vi "WinHostToFlexRIO.vi"() -> ()   [LabVIEW 2013]
doc: "This is the host VI for the 10-Tap 8-Bit Camera with DRAM example. This example demonstrates how to acquire images from a 10-tap, 8-bit, extended configuration, Camera Link camera and display the images on the host. This example supports area scan and line scan cameras for both continuous and finite acquisitions.\n\nThis example also demonstrates the use of DRAM as a frame buffer for very high speed acquisitions. Data packing and flow-control are also employed to maximize use of the available DRAM and FIFOs in terms of both memory space and performance.\n\nAdditionally, the example demonstrates the serial server, which allows third-party camera configuration utilities to communicate with the camera using the Camera Link serial interface while this VI is running."
uses:
  <vilib>/userdefined/High Color/nirio_resource_hc.ctl
  <vilib>/FPGAPlugInAG/PXIe-7966R/niLvFpga_Open_PXIe-7966R.vi
  <vilib>/rvi/interface/common/dynamic/niFpgaDynamicAddResources.vi
  <vilib>/FPGAPlugInAG/Dynamic/niLvFpga_Reset_Dynamic.vi
  <vilib>/rvi/interface/common/niFpgaWaitOnOcc.vi
  <vilib>/Utility/error.llb/Error Cluster From Error Code.vi
  <vilib>/rvi/errors/niLvFpgaAdjustHostInterfaceError.vi
  <vilib>/FPGAPlugInAG/Dynamic/niLvFpga_Run_Dynamic.vi
  <vilib>/LabVIEW Targets/FPGA/FlexRIO/CustomFPGAMethods/79XXR_Method_IOModuleStatusImpl.vi
  <vilib>/FPGAPlugInAG/Dynamic/niLvFpga_Close_Dynamic.vi
  <vilib>/rvi/interface/nirviOpenFPGA/nirviOpenFPGA.xnode
  FPGA Bitfiles/PXIe-7966R_FlexRIOMod1483_8T8_v1_0.lvbitx
  FlexRIO1483_8T8.vi
  <vilib>/rvi/interface/nirviMethod/nirviMethod.xnode
  <vilib>/rvi/interface/nirviReadWriteControl/nirviReadWriteControl.xnode
  <vilib>/rvi/interface/nirviCloseFPGA/nirviCloseFPGA.xnode
  <vilib>/rvi/interface/Simulation/niFpgaSimulationCallBeginRW.vi
  <vilib>/rvi/errors/niLvFpgaMergeErrorWithErrorCode.vi
  <vilib>/FPGAPlugInAG/Dynamic/niLvFpga_ReadFifo_Dynamic.vi
  NiFpgaLv.dll
  <vilib>/FPGAPlugInAG/Dynamic/niLvFpga_ConfigureFifo_Dynamic.vi
  <vilib>/FPGAPlugInAG/Dynamic/niLvFpga_StartFifo_Dynamic.vi
panel:
  out "Frames Received":u32
  out "Error out":errorcluster
  out "Received":bool
  out "Sent":bool
  out "Acquire 3":bool
  out "UART  Received Message":string
  in  "Acquire 2":bool
  in  "UART  Send Message":string
  out "Frame Counter Check":bool
  in  "RIO Device":T1="RIO0"
  out "Ready":bool
  out "Image":T2(plugin-control)
  in  "DAQStartStop":bool
  in  "Stop":bool
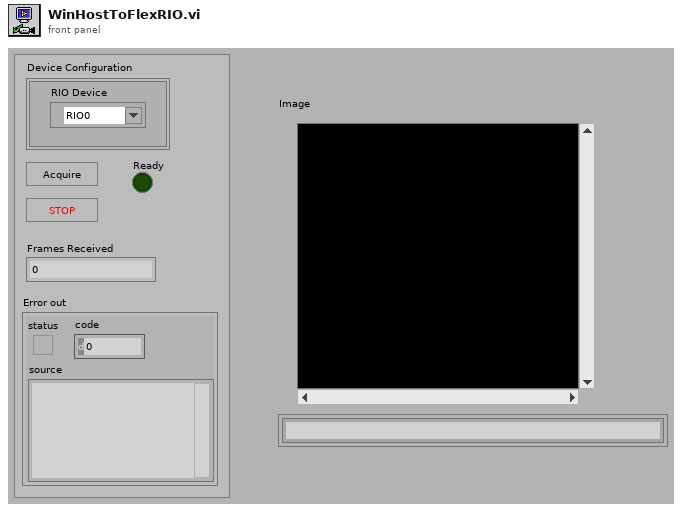
[diagram p1: front panel]
types:
  T1 = typedef "nirio_resource_hc.ctl" = tag
  T2 = typedef "IMAQ Image.ctl" = refnum<image>
  T3 = enum8{"Standard", "Basler 10-tap", "Vosskühler 10-tap"}
  T4 = typedef "Image Type" = u32
  T5 = enum16{"big-endian, network order", "native, host order", "little-endian"}
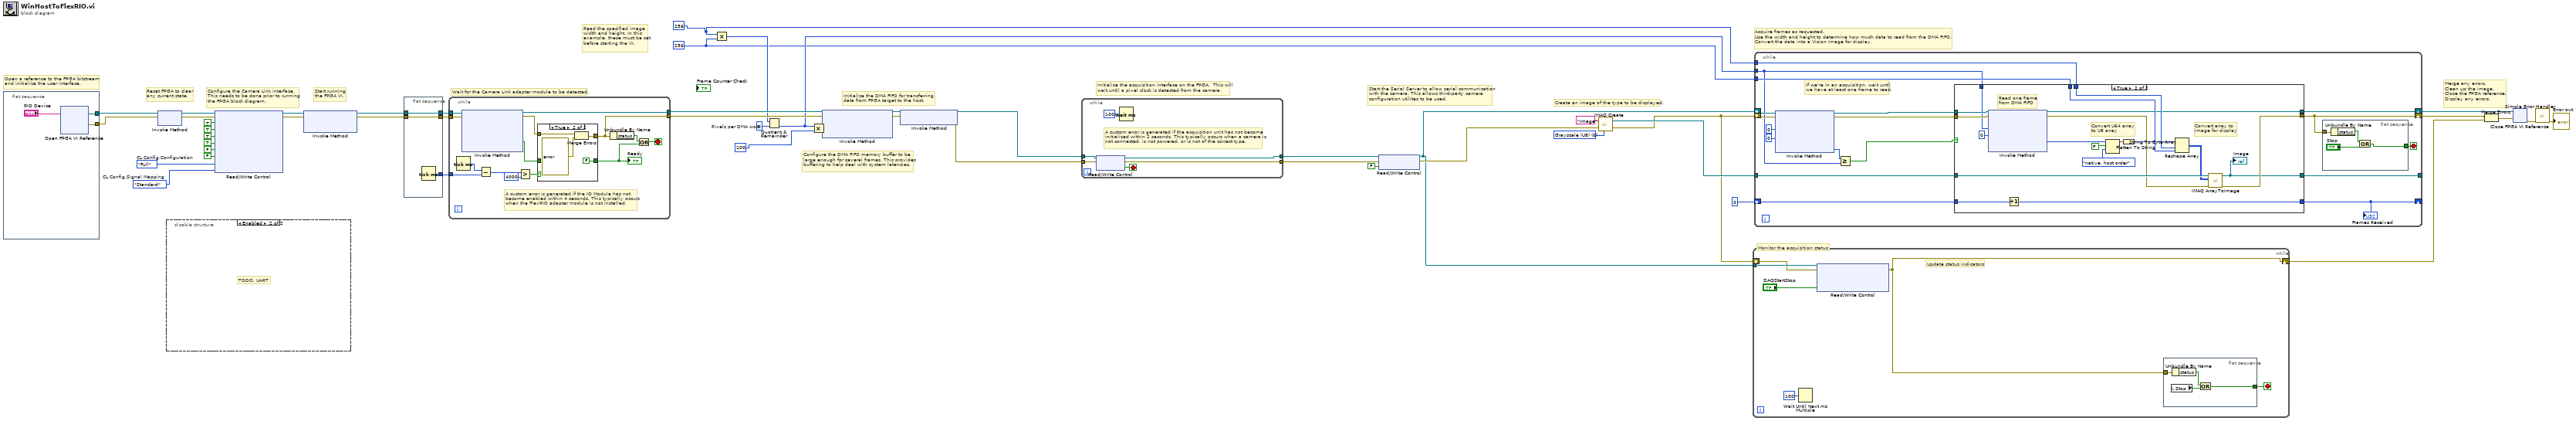
[diagram p0: block diagram]
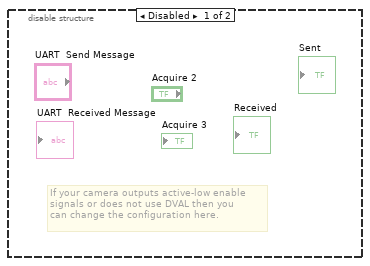
[diagram p2: hidden frame]
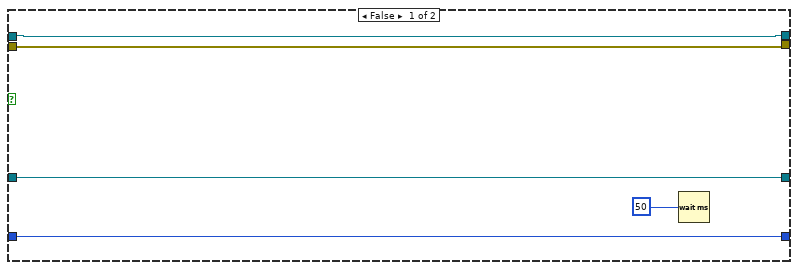
[diagram p3: hidden frame]
diagram:
  w6 = u32 256 ("Image Height")
  w7 = u32 256 ("Image Height")
  w8 = T3."Standard"  # CL Config.Signal Mapping
  w9 = enum8{"Base", "Medium", "Full"}."Full"  # CL Config.Configuration
  w19 = u32 8  # Pixels per DMA word
  w46 = T4 0 items=["Grayscale (U8)", "Grayscale (I16)", "Grayscale (SGL)", "Complex (CSG)", "RGB (U32)", "HSL (U32)", "RGB (U64)", "Grayscale (U16)"] ("Image Type")
  # "Configure the DMA FIFO memory buffer to be\nlarge enough for several frames. This provides\nbuffering to help deal with system latencies."
  # "Start running\nthe FPGA VI."
  # "Reset FPGA to clear\nany current state."
  # "Read the specified image\nwidth and height. In this\nexample, these must be set\nbefore starting the VI."
  # "Merge any errors.\nClean up the image.\nClose the FPGA reference.\nDisplay any errors."
  # "Acquire frames as requested.\nUse the width and height to determine how much data to read from the DMA FIFO.\nConvert the data into a Vision Image for display."
  # "Monitor the acquisition status"
  # "Start the Serial Server to allow serial communication\nwith the camera. This allows third-party camera\nconfiguration utilites to be used."
  # "Create an image of the type to be displayed."
  # "Initialize the acquisition interface on the FPGA.  This will\nwait until a pixel clock is detected from the camera."
  # "Wait for the Camera Link adapter module to be detected."
  # "Initialize the DMA FIFO for transferring\ndata from FPGA target to the host."
  # "Configure the Camera Link interface.\nThis needs to be done prior to running\nthe FPGA block diagram."
  # "Open a reference to the FPGA bitstream\nand initialize the user interface."
  n1 = flat-sequence {
    tunnel: [w50] -> w43
    tunnel: [w49] -> w48
    frame #0 {
      n2 = xnode "Open FPGA VI Reference"("resource name"="RIO Device") -> ("FPGA VI Reference Out"=w50:refnum<k20>, "error out"=w49:errorcluster)  [unwired: 1 in]
    }
  }
  n3 = xnode "Invoke Method"("FPGA VI Reference In"=w43, "error in"=w48) -> ("FPGA VI Reference Out"=w32:refnum<k20>, "error out"=w35:errorcluster)
  n4 = disable-structure shown="Enabled" {
    frame Disabled {
      # "If your camera outputs active-low enable\nsignals or does not use DVAL then you \ncan change the configuration here."
    }
    frame Enabled {
      # "TODO. UART"
    }
  }
  n5 = xnode "Read/Write Control"("FPGA VI Reference In"=w32, "error in"=w35, "FVALHigh"=TRUE ("IO Module Config.CL FVAL Active High"), "LVALHigh"=TRUE ("IO Module Config.CL LVAL Active High"), "DVALHigh"=TRUE ("IO Module Config.CL DVAL Active High"), "SpareHigh"=TRUE ("IO Module Config.CL Spare Active High"), "LineScan"=FALSE, "Acq Control.Ignore DVAL"=FALSE ("CL Config.Line Scan"), "Configuration"=w9, "SignalMapping"=w8) -> ("FPGA VI Reference Out"=w36:refnum<k20>, "error out"=w34:errorcluster)
  n6 = xnode "Invoke Method"("FPGA VI Reference In"=w36, "error in"=w34) -> ("FPGA VI Reference Out"=w22:refnum<k20>, "error out"=w23:errorcluster)  [unwired: 1 in]
  n7 = flat-sequence {
    tunnel: [w54] -> w26
    tunnel: w22 -> [w53]
    tunnel: [w53] -> w25
    tunnel: [w52] -> w24
    tunnel: w23 -> [w52]
    frame #0 {
      n8 = Tick Count (ms)() -> (millisecond timer value=w54:u32)
    }
  }
  n9 = while {
    tunnel: w25 -> [w68]
    tunnel: [w67] -> w42
    tunnel: w24 -> [w66]
    tunnel: [w60] -> w41
    tunnel: w26 -> [w55]
    stop <- w64 stop-if-true
    # "A custom error is generated if the IO Module has not\nbecome enabled within 4 seconds. This typically occurs\nwhen the FlexRIO adapter module is not installed."
    n10 = Tick Count (ms)() -> (millisecond timer value=w58:u32)
    n11 = xnode "Invoke Method"("FPGA VI Reference In"=w68, "error in"=w66) -> ("FPGA VI Reference Out"=w67:refnum<k20>, "error out"=w62:errorcluster, "IO Enabled?"=w59:bool)  [unwired: 3 out]
    n12 = Subtract(x=w58, y=w55) -> (x-y=w57:u32)
    n13 = Greater?(x=w57, y=u32 4000) -> (0:w63:bool)
    n14 = case shown="True" w63 {
      tunnel: [w70 FALSE] -> w61
      tunnel: w59 -> [w70 _]
      tunnel: w62 -> [w69 w72]
      tunnel: [w69 w74] -> w60
      frame False {
      }
      frame True {
        n15 = Merge Errors(w72, errorcluster {"status"=TRUE, "code"=-8999, "source"="IO Module Status: The IO Module did not initialize before the specified timeout. This typically occurs when the FlexRIO adapter module is not properly connected to the FlexRIO FPGA module."} ("error in")) -> (w74:errorcluster)
      }
    }
    "Ready" <- w61
    n16 = Unbundle By Name(w60) -> ("status"=w65:bool)
    n17 = Or(x=w65, y=w61) -> (x .or. y?=w64:bool)
  }
  n18 = Multiply(x=w7, y=w6) -> (x*y=w18:u32)
  n19 = Quotient & Remainder(x=w18, y=w19) -> (floor(x/y)=w17:u32)  [unwired: 1 out]
  n20 = Multiply(x=w17, y=u32 100 ("Image Height")) -> (x*y=w27:u32)
  n21 = xnode "Invoke Method"("FPGA VI Reference In"=w42, "error in"=w41, "Requested Depth"=w27) -> ("FPGA VI Reference Out"=w40:refnum<k20>, "error out"=w39:errorcluster)  [unwired: 1 out]
  n22 = xnode "Invoke Method"("FPGA VI Reference In"=w40, "error in"=w39) -> ("FPGA VI Reference Out"=w16:refnum<k20>, "error out"=w15:errorcluster)
  n23 = while {
    tunnel: w16 -> [w79]
    tunnel: w15 -> [w78]
    tunnel: [w76] -> w13
    tunnel: [w75] -> w12
    stop <- w77 stop-if-true
    # "A custom error is generated if the acquisition unit has not become\ninitialized within 2 seconds. This typically occurs when a camera is\nnot connected, is not powered, or is not of the correct type."
    n24 = xnode "Read/Write Control"("FPGA VI Reference In"=w79, "error in"=w78) -> ("FPGA VI Reference Out"=w76:refnum<k20>, "error out"=w75:errorcluster, "InitDone"=w77:bool)
    n25 = Wait (ms)(milliseconds to wait=u32 100) -> ()  [unwired: 1 out]
  }
  n26 = xnode "Read/Write Control"("FPGA VI Reference In"=w13, "error in"=w12, "DAQStartStop"=FALSE) -> ("FPGA VI Reference Out"=w1:refnum<k20>, "error out"=w11:errorcluster)
  n27 = call "IMAQ Create"("Image Name"="Image", "Image Type"=w46, "error in (no error)"=w11) -> ("New Image"=w20:T2, "error out"=w2:errorcluster)  [unwired: 2 in]
  n28 = while {
    tunnel: w1 -> [w83]
    shift-right: [w86] -> w37
    shift-left: w2 -> [w81]
    stop <- w85 stop-if-true
    # "Update status indicators"
    n29 = Wait Until Next ms Multiple(millisecond multiple=u32 100) -> ()  [unwired: 1 out]
    n30 = xnode "Read/Write Control"("FPGA VI Reference In"=w83, "error in"=w81, "DAQStartStop"="DAQStartStop") -> ("error out"=w86:errorcluster)  [unwired: 3 out]
    n31 = flat-sequence {
      tunnel: w86 -> [w90]
      tunnel: [w88] -> w85
      frame #0 {
        n32 = local read "Stop"() -> (w87:bool)
        n33 = Unbundle By Name(w90) -> ("status"=w89:bool)
        n34 = Or(x=w89, y=w87) -> (x .or. y?=w88:bool)
      }
    }
  }
  n35 = while {
    tunnel: w17 -> [w92]
    tunnel: w7 -> [w108]
    tunnel: w6 -> [w107]
    tunnel: w20 -> [w106]
    tunnel: [w102] -> _
    shift-right: [w101] -> _
    shift-left: u32 0 -> [w100]
    shift-right: [w105] -> w45
    shift-left: w1 -> [w99]
    shift-right: [w104] -> w38
    shift-left: w2 -> [w98]
    stop <- w103 stop-if-true
    # "If we're in an acquisition, wait until\nwe have at least one frame to read."
    n36 = xnode "Invoke Method"("FPGA VI Reference In"=w99, "error in"=w98, "Number of Elements"=u32 0, "Timeout (ms)"=0) -> ("FPGA VI Reference Out"=w97:refnum<k20>, "error out"=w96:errorcluster, "Elements Remaining"=w93:u32)  [unwired: 1 out]
    n37 = Greater Or Equal?(x=w93, y=w92) -> (x >= y?=w91:bool)
    n38 = case shown="True" w91 {
      tunnel: w92 -> [_ w124]
      tunnel: w108 -> [_ w136]
      tunnel: w107 -> [_ w135]
      tunnel: w106 -> [w117 w134]
      tunnel: [w114 w132] -> w104
      tunnel: [w115 w131] -> w105
      tunnel: [w117 w118] -> w102
      tunnel: w100 -> [w116 w130]
      tunnel: [w116 w129] -> w101
      tunnel: w97 -> [w115 w127]
      tunnel: w96 -> [w114 w126]
      frame False {
        n39 = Wait (ms)(milliseconds to wait=u32 50 ("millisecond multiple")) -> ()  [unwired: 1 out]
      }
      frame True {
        # "Convert U64 array\nto U8 array"
        # "Convert array to\nimage for display"
        # "Read one frame\nfrom DMA FIFO"
        n40 = xnode "Invoke Method"("FPGA VI Reference In"=w127, "error in"=w126, "Number of Elements"=w124, "Timeout (ms)"=0) -> ("FPGA VI Reference Out"=w131:refnum<k20>, "error out"=w133:errorcluster, "Data"=w128:u64[])  [unwired: 1 out]
        n41 = Increment(x=w130) -> (x+1=w129:u32)
        n42 = Flatten To String(anything=w128, prepend array or string size? (T)=FALSE, byte order (0:big-endian, network order)=T5."native, host order") -> (data string=w120:string)  [unwired: 1 in, 2 out]
        n43 = String To Byte Array(string=w120) -> (unsigned byte array=w119:u8[])
        n44 = Reshape Array(w119, w136, w135) -> (w123:u8[][])
        n45 = call "IMAQ ArrayToImage"("error in (no error)"=w133, "Image Pixels (U8)"=w123, "Image"=w134) -> ("error out"=w132:errorcluster, "Image Out"=w118:T2)  [unwired: 7 in]
        "Image" <- w118
      }
    }
    "Frames Received" <- w101
    n46 = flat-sequence {
      tunnel: w104 -> [w110]
      tunnel: [w109] -> w103
      frame #0 {
        n47 = Unbundle By Name(w110) -> ("status"=w111:bool)
        n48 = Compound Arithmetic op=OR(w111, "Stop") -> (w109:bool)
      }
    }
  }
  n49 = Merge Errors(w38, w37) -> (w14:errorcluster)
  n50 = xnode "Close FPGA VI Reference"("FPGA VI Reference In"=w45, "error in"=w14) -> ("error out"=w44:errorcluster)
  n51 = call <vilib>:"Simple Error Handler.vi"("error in (no error)"=w44) -> ("error out"=→"Error out":errorcluster)  [unwired: 4 in, 4 out]
